vi "main.vi"() -> ()   [LabVIEW 2023]
doc: "Purpose:\n\nThis VI (Virtual Instrument) generates a sequence of random values between -0.5 and 0.5, and calculates the moving average over the last 8 generated values. The mean value is displayed in real-time, providing a continuously updated average as new values are generated.\n\nComponents:\n\nRandom Value Generator:\n- Generates random numbers between -0.5 and 0.5 on each iteration.\nShift Register:\n-Holds an array of the last 8 random values. Each new random value replaces the oldest one, ensuring that only the 8 most recent values are stored at any time.\nSum Calculation:\n-The values in the shift register are summed to provide the total of the last 8 values.\nMean Calculation:\n-The sum is divided by 8 (the number of values in the shift register) to calculate the moving average.\nMean Value Indicator:\n-Displays the calculated mean value in real-time.\nLoop Timer:\n-Sets the delay between each iteration of the loop (200 ms), controlling the rate of random value generation and mean calculation.\nStop Button:\n-Allows the user to stop the VI execution.\n\nUsage:\n\nStart the VI to begin generating random values and calculating their moving average.\nThe Mean Value Indicator will update every 200 ms, showing the current average of the last 8 random values.\nUse the Stop Button to end the VI execution."
uses:
  <vilib>/numeric/Random Number (Range) DBL.vi
panel:
  out "Mean value indicator":cluster{"number":dbl, dbl}(graph)
  in  "?":bool
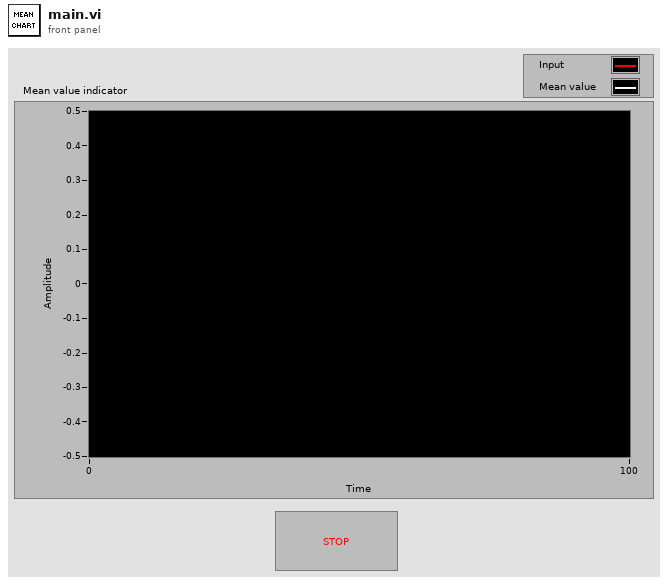
[diagram p1: front panel]
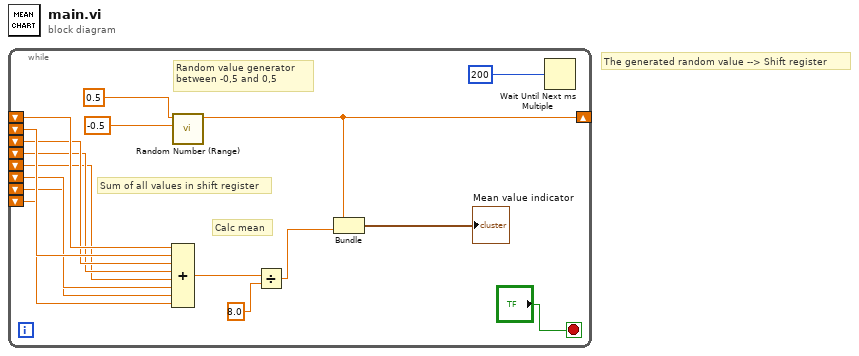
[diagram p0: block diagram]
diagram:
  # "The generated random value --> Shift register"
  n1 = while {
    shift-right: [w13] -> _
    shift-left: _ -> [w12]
    shift-left: _ -> [w11]
    shift-left: _ -> [w10]
    shift-left: _ -> [w9]
    shift-left: _ -> [w8]
    shift-left: _ -> [w7]
    shift-left: _ -> [w6]
    shift-left: _ -> [w5]
    stop <- "?" stop-if-true
    # "Calc mean"
    # "Sum of all values in shift register"
    # "Random value generator  \nbetween -0,5 and 0,5"
    n2 = Compound Arithmetic op=ADD(w12, w11, w10, w9, w8, w7, w6, w5) -> (w4:dbl)
    n3 = call-poly <vilib>:"Random Number (Range).vi"("lower bound (0)"=-0.5, "upper bound (100)"=0.5) -> ("number"=w13:dbl)  [unwired: 9 in]
    n4 = Divide(x=w4, y=8.0) -> (x/y=w2:dbl)
    n5 = Bundle("number"=w13, w2) -> (→"Mean value indicator":cluster{"number":dbl, dbl})  [unwired: 1 in]
    n6 = Wait Until Next ms Multiple(millisecond multiple=u32 200 ("millisecond timer value")) -> ()  [unwired: 1 out]
  }
